vi "Handle Command.vi"(8 "error in (no error)":errorcluster, 9 "Data":variant, 10 "Command":string, 11 "Inst.TC in":refnum<class "Inst.TC.lvclass">) -> (0 "error out":errorcluster, 1 "Processed Data":variant, 2 "Command":string, 3 "Inst.TC out":refnum<class "Inst.TC.lvclass">)   [LabVIEW 2019, in "Inst.TC.lvclass"]
uses:
  Inst.TC.lvclass
  Typedefs/Inst.TC.Commands--Enum.ctl
  <userlib>/LevyLab/Instrument Framework/Instrument Types/Cryostat/Typedefs/getHeater--cluster.ctl
  Inst.TC.lvclass/Inst.TC.ctl
  <userlib>/LevyLab/Instrument Framework/Instrument Types/Cryostat/Typedefs/getTemperature--cluster.ctl
  58991851-e4f0-4ee5-bf4a-dfca5dd48c95.vi
  1e1ed493-89ac-4a60-b33b-3a503c3fd0e1.vi
  58991851-e4f0-4ee5-bf4a-dfca5dd48c95.vi/4143c617-15f4-47e8-afad-989cfea312de.vi
  58991851-e4f0-4ee5-bf4a-dfca5dd48c95.vi/06f712b7-eed4-462a-a582-f657c6ba0d49.vi
  1e1ed493-89ac-4a60-b33b-3a503c3fd0e1.vi/15136f2d-002b-4be8-a771-2a1a2e179ae4.vi
  1e1ed493-89ac-4a60-b33b-3a503c3fd0e1.vi/0fcc48dd-7f95-46e4-8112-87f244fbf0c6.vi
  <vilib>/Utility/Data Type/Get Type Information.vi
  <vilib>/JDP Science/JSONtext/JSON text to Variant.vi
  <vilib>/JDP Science/JSONtext/LVClass Serializer/JSONtext LVClass Serializer.lvclass
  <userlib>/LevyLab/Instrument Framework/Instrument Types/Cryostat/Instrument.Cryostat.lvclass
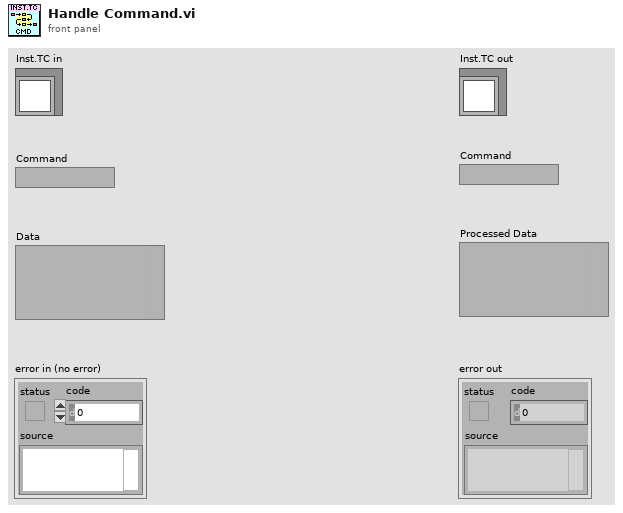
[diagram p1: front panel]
types:
  T1 = typedef "Instrument.Cryostat.lvclass/getHeater--cluster.ctl" = cluster{"current":dbl, "status":string}
  T2 = typedef "Instrument.Cryostat.lvclass/getTemperature--cluster.ctl" = cluster{"temperature":dbl, "status":string, "finished":bool}
  T3 = typedef "Inst.TC.lvclass/Inst.TC.Commands--Enum.ctl" = enum16{"getTemperature", "getHeater", "setHeater"}
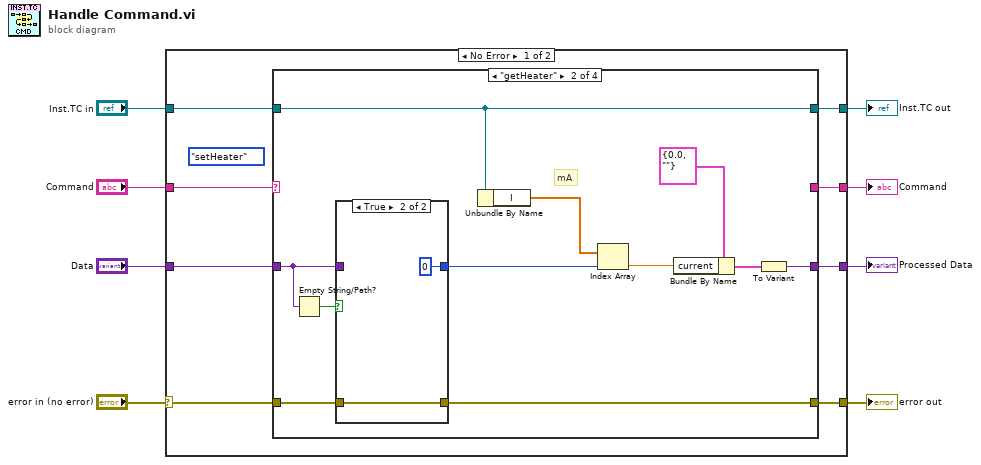
[diagram p0: block diagram]
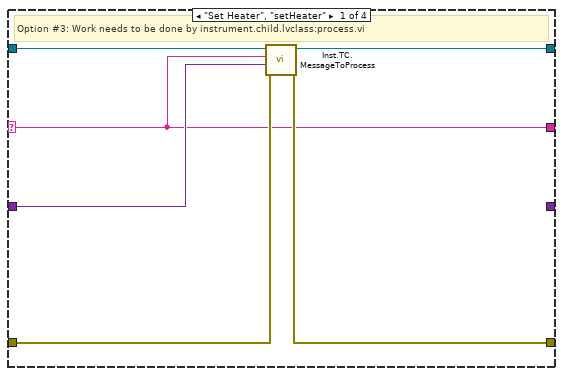
[diagram p2: hidden frame]
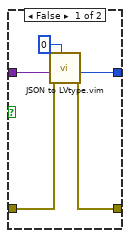
[diagram p3: hidden frame]
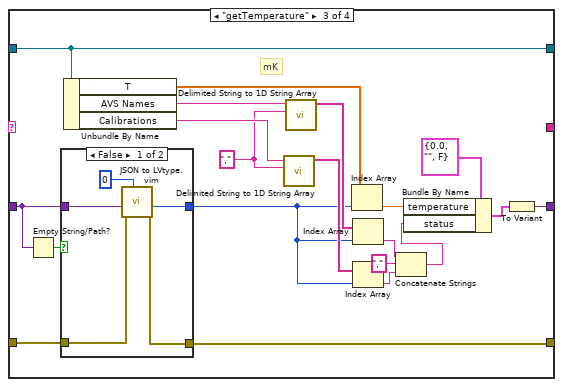
[diagram p4: hidden frame]
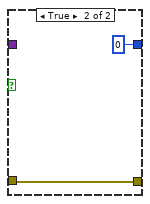
[diagram p5: hidden frame]
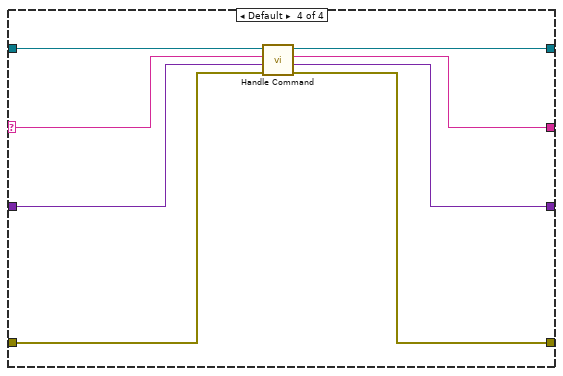
[diagram p6: hidden frame]
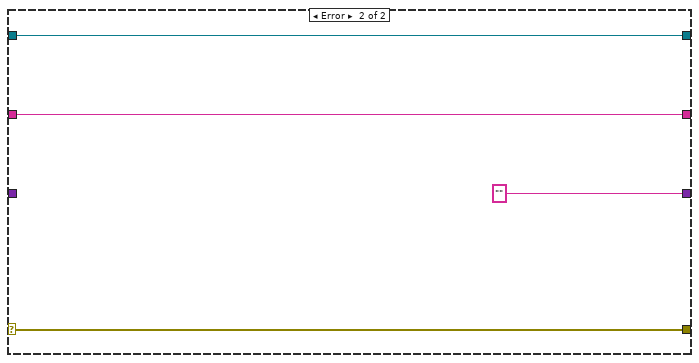
[diagram p7: hidden frame]
diagram:
  n1 = case shown="No Error" "error in (no error)" {
    selector: "error in (no error)" -> [w10 w79]
    tunnel: [w12 w79] -> w6
    tunnel: [w14 w78] -> w5
    tunnel: "Inst.TC in" -> [w15 w78]
    tunnel: "Command" -> [w16 w76]
    tunnel: [w13 "" ("String")] -> w3
    tunnel: "Data" -> [w9 _]
    tunnel: [w11 w76] -> w1
    frame No Error {
      (unwired) Inst.TC.Commands--Enum."setHeater" ("Commands")
      n2 = case shown="\"getHeater\"" w16 {
        selector: w16 -> [w17 _ _ w69]
        tunnel: w15 -> [w22 w32 w58 w73]
        tunnel: [w21 w32 w58 w70] -> w14
        tunnel: [_ w33 w59 w72] -> w13
        tunnel: w10 -> [w20 w31 w57 w74]
        tunnel: w9 -> [w18 w25 w43 w75]
        tunnel: [w19 w30 w56 w71] -> w12
        tunnel: [w17 _ _ w68] -> w11
        frame "Set Heater", "setHeater" {
          # "Option #3: Work needs to be done by instrument.child.lvclass:process.vi"
          n3 = call "Inst.TC.MessageToProcess.vi"("error in (no error)"=w20, "Data"=w18, "Command"=w17, "Inst.TC in"=w22) -> ("error out"=w19:errorcluster, "Inst.TC out"=w21:refnum<class "Inst.TC.lvclass">)  [unwired: 6 in]
        }
        frame "getHeater" {
          # "mA"
          n4 = Empty String/Path?(string/path=w25) -> (empty?=w24:bool)
          n5 = case shown="True" w24 {
            tunnel: w25 -> [w38 _]
            tunnel: w31 -> [w37 w39]
            tunnel: [w36 w39] -> w30
            tunnel: [w35 0 ("Data out")] -> w29
            frame False {
              n6 = call "JSON to LVtype.vim"("type"=0, "error in (no error)"=w37, "JSON Data in"=w38) -> ("error out"=w36:errorcluster, "Data out"=w35:i32)  [unwired: 7 in]
            }
            frame True {
            }
          }
          n7 = Unbundle By Name(w32) -> ("I"=w23:dbl[])
          n8 = Index Array(array=w23, index=w29) -> (element=w26:dbl)
          n9 = Bundle By Name(cluster=T1 {"current"=0.0, "status"=""} ("getHeat"), "current"=w26) -> (w27:T1)
          n10 = To Variant(anything=w27) -> (Variant=w33:variant)
        }
        frame "getTemperature" {
          w51 = "," ("delimiter")
          # "mK"
          n11 = Empty String/Path?(string/path=w43) -> (empty?=w42:bool)
          n12 = case shown="False" w42 {
            tunnel: w43 -> [w65 _]
            tunnel: w57 -> [w64 w67]
            tunnel: [w63 w67] -> w56
            tunnel: [w61 0 ("Data out")] -> w44
            frame False {
              n13 = call "JSON to LVtype.vim"("type"=0, "error in (no error)"=w64, "JSON Data in"=w65) -> ("error out"=w63:errorcluster, "Data out"=w61:i32)  [unwired: 7 in]
            }
            frame True {
            }
          }
          n14 = Unbundle By Name(w58) -> ("T"=w60:dbl[], "AVS Names"=w53:string, "Calibrations"=w52:string)
          n15 = call <vilib>:"Delimited String to 1D String Array.vi"("delimiter"=w51, "delimited string"=w52) -> ("string array"=w50:string[])  [unwired: 9 in]
          n16 = call <vilib>:"Delimited String to 1D String Array.vi"("delimiter"=w51, "delimited string"=w53) -> ("string array"=w49:string[])  [unwired: 9 in]
          n17 = Index Array(array=w60, index=w44) -> (element=w41:dbl)
          n18 = Index Array(array=w49, index=w44) -> (element=w48:string)
          n19 = Index Array(array=w50, index=w44) -> (element=w47:string)
          n20 = Concatenate Strings(w48, "," ("string"), w47) -> (w45:string)
          n21 = Bundle By Name(cluster=T2 {"temperature"=0.0, "status"="", "finished"=FALSE} ("getTemperature"), "temperature"=w41, "status"=w45) -> (w54:T2)
          n22 = To Variant(anything=w54) -> (Variant=w59:variant)
        }
        frame Default {
          n23 = call-parent "Handle Command.vi"("error in (no error)"=w74, "params in"=w75, "command"=w69, "Instrument in"=w73) -> ("error out"=w71:errorcluster, "processed data"=w72:variant, "command out"=w68:string, "Instrument out"=w70:refnum<class "Inst.TC.lvclass">)  [unwired: 4 in]
        }
      }
    }
    frame Error {
    }
  }
  "error out" <- w6
  "Inst.TC out" <- w5
  "Command" <- w1
  "Processed Data" <- w3
